vi "powermeter-start.vi"(8 "error in (no error)":errorcluster, 11 "Powermeter":refnum<vi>) -> (0 "error out":errorcluster, 3 "Powermeter OUT":refnum<vi>)   [LabVIEW 2016]
uses:
  controls/powermeter.ctl
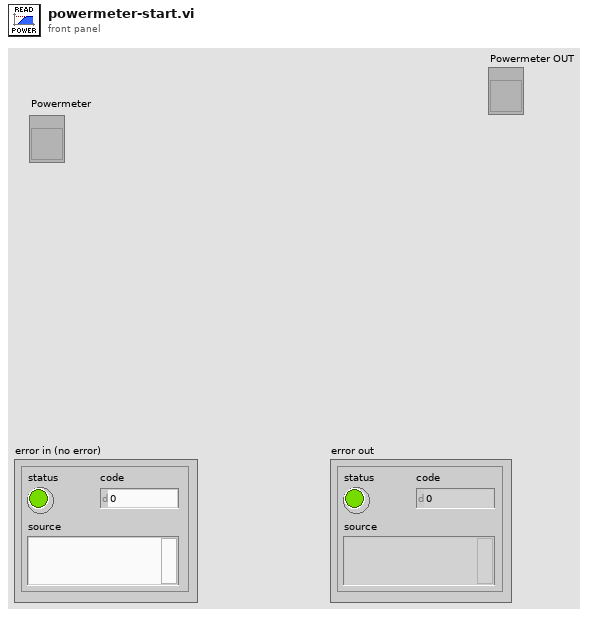
[diagram p1: front panel]
types:
  T1 = typedef "powermeter.ctl" = cluster{"Start":bool, "Serial ":string, "Model":string, "Sensor":string, "Power":dbl, "Density":bool, "Lambda":dbl, "Open":bool, "Save":bool, "reference":refnum<k7>, "hDevice":i32, "Dev. Std.":dbl, "Channel":i16}
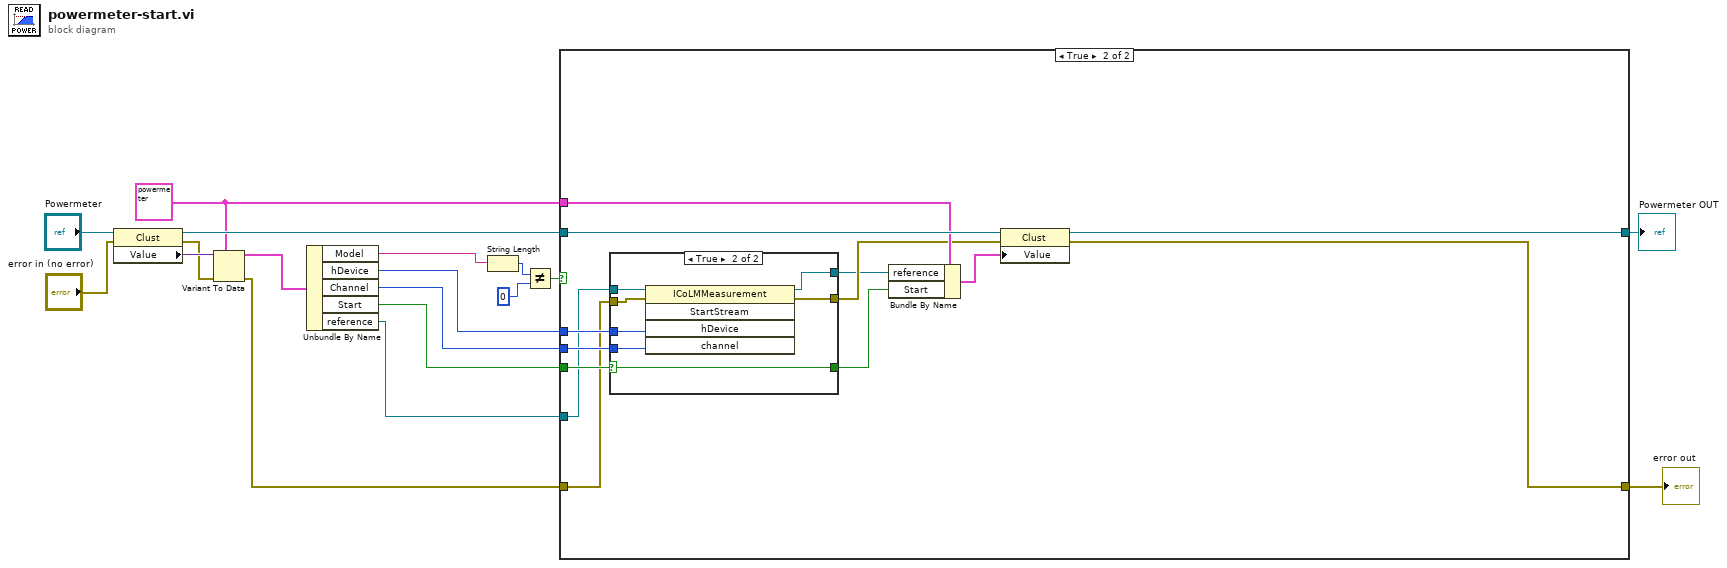
[diagram p0: block diagram]
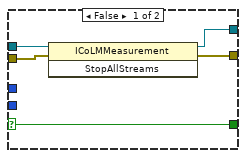
[diagram p3: hidden frame]
diagram:
  w2 = T1 {"Start"=FALSE, "Serial "="", "Model"="", "Sensor"="", "Power"=0.0, "Density"=FALSE, "Lambda"=0.0, "Open"=FALSE, "Save"=FALSE, "reference"=refnum, "hDevice"=0, "Dev. Std."=0.0, "Channel"=0} ("Power Meter")
  n1 = property class="Clust"(reference="Powermeter", error in="error in (no error)") -> (reference out=w4:refnum<vi>, error out=w16:errorcluster, "Value"=w17:variant)
  n2 = Variant To Data(error in=w16, type=w2, Variant=w17) -> (data=w14:T1, error out=w12:errorcluster)
  n3 = Unbundle By Name(w14) -> ("Model"=w11:string, "hDevice"=w7:i32, "Channel"=w6:i16, "Start"=w5:bool, "reference"=w3:refnum<k7>)
  n4 = String Length(string=w11) -> (length=w10:i32)
  n5 = Not Equal?(x=w10, y=0) -> (x != y?=w8:bool)
  n6 = case shown="True" w8 {
    tunnel: w12 -> [w20 w29]
    tunnel: [w20 w24] -> w18
    tunnel: w7 -> [_ w33]
    tunnel: w6 -> [_ w32]
    tunnel: w5 -> [_ w31]
    tunnel: w4 -> [w19 w28]
    tunnel: w3 -> [_ w30]
    tunnel: w2 -> [_ w27]
    tunnel: [w19 w21] -> w1
    frame False {
    }
    frame True {
      n7 = case shown="True" w31 {
        selector: w31 -> [w34 w39]
        tunnel: w33 -> [_ w45]
        tunnel: w32 -> [_ w44]
        tunnel: [w36 w43] -> w25
        tunnel: w30 -> [w38 w42]
        tunnel: w29 -> [w37 w41]
        tunnel: [w35 w40] -> w23
        tunnel: [w34 w39] -> w22
        frame False {
          n8 = invoke class="ICoLMMeasurement" method="StopAllStreams"(reference=w38, error in=w37) -> (reference out=w35:refnum<k7>, error out=w36:errorcluster)  [unwired: 1 in, 1 out]
        }
        frame True {
          n9 = invoke class="ICoLMMeasurement" method="StartStream"(reference=w42, error in=w41, "hDevice"=w45, "channel"=w44) -> (reference out=w40:refnum<k7>, error out=w43:errorcluster)  [unwired: 1 in, 3 out]
        }
      }
      n10 = Bundle By Name(cluster=w27, "reference"=w23, "Start"=w22) -> (w26:T1)
      n11 = property class="Clust"(reference=w28, error in=w25, "Value"=w26) -> (reference out=w21:refnum<vi>, error out=w24:errorcluster)
    }
  }
  "error out" <- w18
  "Powermeter OUT" <- w1
